vi "Create External Network Step Reference.vi"(8 "error in (no error)":errorcluster, 11 "QPA Measurement in":refnum<class "QPA Measurement.lvclass">) -> (0 "error out":errorcluster, 3 "QPA Measurement out":refnum<class "QPA Measurement.lvclass">)   [LabVIEW 2016, in "QPA Measurement.lvlib" / "QPA Measurement.lvclass"]
uses:
  QPA Measurement.lvclass
  C:/Projects/STS/Common/Sequence Automation/Plugins/Measurement Interface.lvlibp/Measurement Interface.lvclass
  QPA Measurement.lvclass/QPA Measurement.ctl
  Plugins/Measurement Interface.lvlibp/Private Methods/Engine Reference/Read Engine Reference.vi
  Plugins/Measurement Interface.lvlibp/Private Methods/Active Sequence File/Read Active Sequence File.vi
  Plugins/TestStand API Tools (TSAT).lvlibp/Step Actions/TSAT Step Actions.lvlib
  Plugins/TestStand API Tools (TSAT).lvlibp/Sequence File Actions/TSAT Sequence File Actions.lvlib
  Plugins/TestStand API Tools (TSAT).lvlibp/Sequence Actions/TSAT Sequence Actions.lvlib
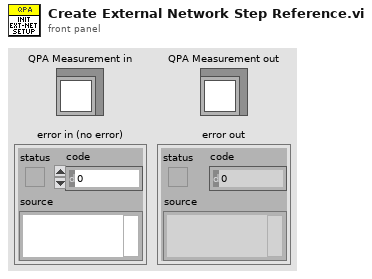
[diagram p1: front panel]
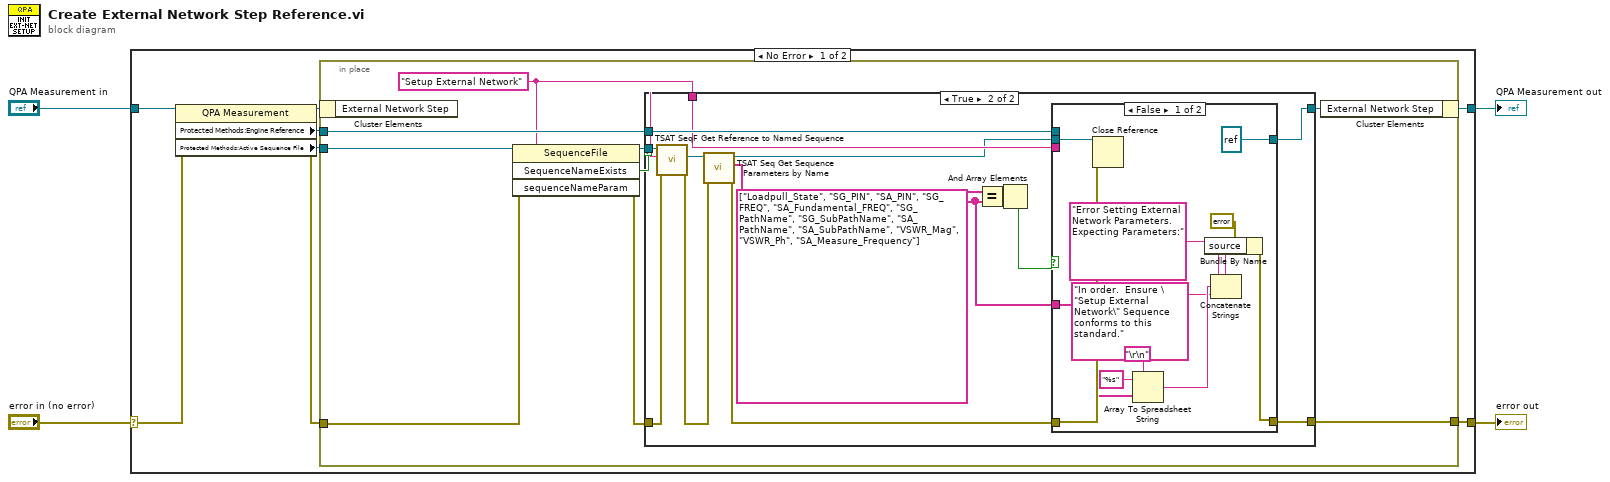
[diagram p0: block diagram]
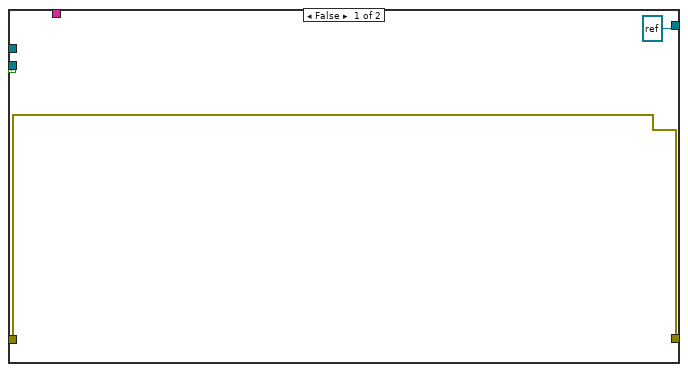
[diagram p2: hidden frame]
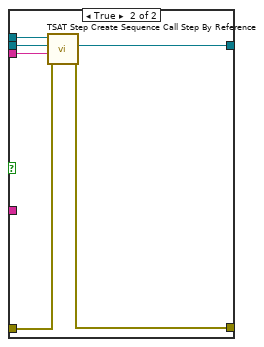
[diagram p3: hidden frame]
diagram:
  n1 = case shown="No Error" "error in (no error)" {
    selector: "error in (no error)" -> [w11 w57]
    tunnel: [w7 w57] -> w3
    tunnel: [w12 w56] -> w1
    tunnel: "QPA Measurement in" -> [w10 w56]
    frame No Error {
      n2 = property class="QPA Measurement"(reference=w10, error in=w11) -> (reference out=w9:refnum<class "QPA Measurement.lvclass">, error out=w5:errorcluster, "Protected Methods:Engine Reference"=w8:refnum<k7>, "Protected Methods:Active Sequence File"=w6:refnum<k7>)
      n3 = in-place {
        in-place-border: w5 -> [w18]
        in-place-border: w8 -> [w21]
        in-place-border: [w20] -> w7
        in-place-border: w6 -> [w16]
        w14 = "Setup External Network" ("Step Name")
        n4 = in-place-cluster #1(w9) -> ()  [unwired: 1 out]
        n5 = invoke class="SequenceFile" method="SequenceNameExists"(reference=w16, error in=w18, "sequenceNameParam"=w14) -> (reference out=w15:refnum<k7>, error out=w17:errorcluster, "SequenceNameExists"=w13:bool)  [unwired: 1 in, 1 out]
        n6 = case shown="True" w13 {
          tunnel: w21 -> [_ w37]
          tunnel: [w22 w36] -> w20
          tunnel: [refnum<k7> refnum ("Step Reference") w35] -> w19
          tunnel: w17 -> [w22 w34]
          tunnel: w15 -> [_ w33]
          tunnel: w14 -> [_ w32]
          frame False {
          }
          frame True {
            w24 = string[] ["Loadpull_State", "SG_PIN", "SA_PIN", "SG_FREQ", "SA_Fundamental_FREQ", "SG_PathName", "SG_SubPathName", "SA_PathName", "SA_SubPathName", "VSWR_Mag", "VSWR_Ph", "SA_Measure_Frequency"] ("y")
            n7 = call "TSAT SeqF Get Reference to Named Sequence.vi"("Error In"=w34, "Seqeunce to Retrieve"=w32, "Sequence File In"=w33) -> ("Error Out"=w29:errorcluster, "Named Sequence"=w31:refnum<k7>)  [unwired: 6 in, 1 out]
            n8 = call "TSAT Seq Get Sequence Parameters by Name.vi"("Error In"=w29, "Sequence Reference In"=w31) -> ("Error Out"=w28:errorcluster, "SubProperty Names"=w27:string[], "Sequence Reference Out"=w30:refnum<k7>)  [unwired: 7 in]
            n9 = Equal?(x=w27, y=w24) -> (x = y?=w26:bool[])
            n10 = And Array Elements(Boolean array=w26) -> (logical AND=w25:bool)
            n11 = case shown="False" w25 {
              tunnel: w37 -> [_ w55]
              tunnel: [w38 w54] -> w36
              tunnel: [refnum<k7> refnum ("Step Reference") w53] -> w35
              tunnel: w32 -> [_ w52]
              tunnel: w30 -> [w49 w51]
              tunnel: w28 -> [w48 w50]
              tunnel: w24 -> [w45 _]
              frame False {
                n12 = Close Reference(reference=w49, error in (no error)=w48) -> ()  [unwired: 1 out]
                n13 = Array To Spreadsheet String(delimiter (Tab)="\r\n", array=w45, 3:"%s" ("format string")) -> (spreadsheet string=w41:string)
                n14 = Concatenate Strings("Error Setting External Network Parameters.  Expecting Parameters:", w41, "In order.  Ensure \"Setup External Network\" Sequence conforms to this standard.") -> (w39:string)
                n15 = Bundle By Name(cluster=errorcluster {"status"=TRUE, "code"=7101, "source"=""} ("error constant"), "source"=w39) -> (w38:errorcluster)
              }
              frame True {
                n16 = call "TSAT Step Create Sequence Call Step By Reference.vi"("Error In"=w50, "Step Name"=w52, "Sequence to Call"=w51, "Engine In"=w55) -> ("Error Out"=w54:errorcluster, "Step Reference"=w53:refnum<k7>)  [unwired: 5 in, 1 out]
              }
            }
          }
        }
        n17 = in-place-cluster #1("External Network Step"=w19) -> (w12:refnum<class "QPA Measurement.lvclass">)
      }
    }
    frame Error {
    }
  }
  "error out" <- w3
  "QPA Measurement out" <- w1
